vi "Ignore Specific Errors.vi"(8 "error in (no error)":errorcluster, 11 "Array":i32[](array[numeric])) -> (0 "error out":errorcluster, 2 "In List?":bool)   [LabVIEW 2019]
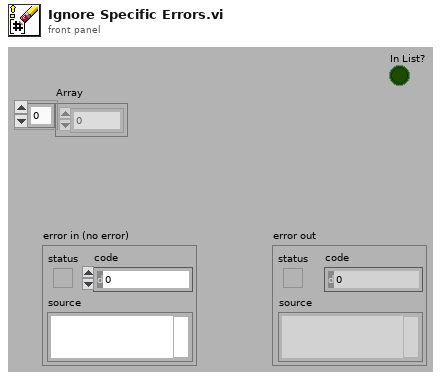
[diagram p1: front panel]
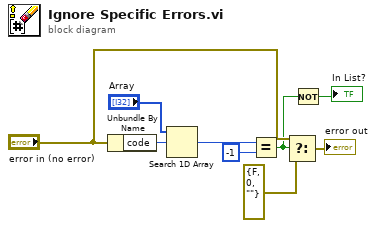
[diagram p0: block diagram]
diagram:
  n1 = Unbundle By Name("error in (no error)") -> ("code"=w9:i32)
  n2 = Search 1D Array(1D array="Array", element=w9) -> (index of element=w7:i32)  [unwired: 1 in]
  n3 = Equal?(x=w7, y=-1) -> (x = y?=w2:bool)
  n4 = Select(t="error in (no error)", s=w2, f=errorcluster {"status"=FALSE, "code"=0, "source"=""}) -> (s? t:f=→"error out":errorcluster)
  n5 = Not(x=w2) -> (.not. x?=→"In List?":bool)
